vi "Parse QD Input.vi"(10 "QD window text":string, 11 "Shift Pressed?":bool) -> (3 "Element to show log for":string)   [LabVIEW 2018, in "TortoiseGit Show Log.lvlib"]
doc: "Looks at what has been typed into the QuickDrop Window. If shift is pressed, this VI always assumes it is the folder and ignores what is entered. Blank compares files. Otherwise, parse the text typed into the wWindow."
uses:
  TortoiseGit Show Log.lvlib
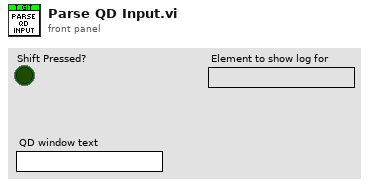
[diagram p1: front panel]
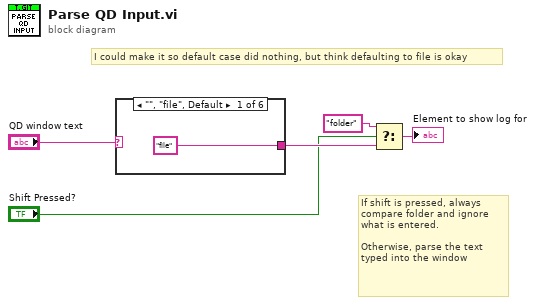
[diagram p0: block diagram]
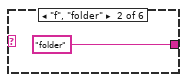
[diagram p2: hidden frame]
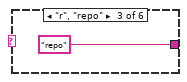
[diagram p3: hidden frame]
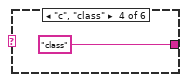
[diagram p4: hidden frame]
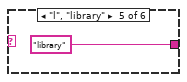
[diagram p5: hidden frame]
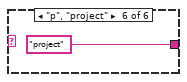
[diagram p6: hidden frame]
diagram:
  # "I could make it so default case did nothing, but think defaulting to file is okay"
  # "If shift is pressed, always compare folder and ignore what is entered.\n\nOtherwise, parse the text typed into the window"
  n1 = case shown="\"\", \"file\", Default" "QD window text" {
    tunnel: ["file" "folder" "repo" "class" "library" "project"] -> w4
    frame "", "file", Default {
    }
    frame "f", "folder" {
    }
    frame "r", "repo" {
    }
    frame "c", "class" {
    }
    frame "l", "library" {
    }
    frame "p", "project" {
    }
  }
  n2 = Select(t="folder" ("Value"), s="Shift Pressed?", f=w4) -> (s? t:f=→"Element to show log for":string)
